vi "PicoScope2000GetTimebase2.vi"(4 "Number of Samples":u32, 6 "Memory Segment":u32, 7 "Acquisition Settings":T2 {"postTriggerSamples" format="%_6p"; "preTriggerSamples" format="%_6p"}, 10 "handle in":i16, 11 "error in (no error)":errorcluster) -> (2 "handle out":i16, 3 "error out":errorcluster, 5 "Properties Panel":T1 {"Max Total Capture Time Available (sec)" format="%.3p"; "Sample Frequency" format="%.3p"; "Sample Rate" format="%.3p"; "Max Samples Available" format="%.3p"; "Total Capture Time (sec)" format="%.3p"})   [LabVIEW 2009]
uses:
  ps2000.dll
  shared/Acquisition Settings.ctl
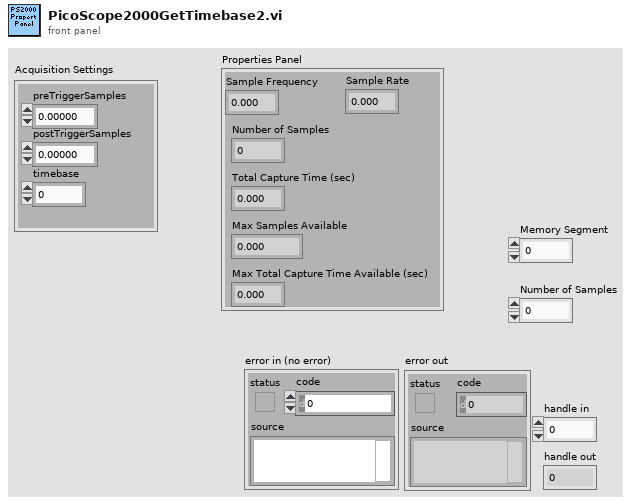
[diagram p1: front panel]
types:
  T1 = cluster{"Sample Frequency":sgl, "Sample Rate":sgl, "Max Samples Available":i32, "Number of Samples":u32, "Total Capture Time (sec) ":sgl, "Max Total Capture Time Available (sec)":sgl}
  T2 = typedef "Acquisition Settings.ctl" = cluster{"preTriggerSamples":u64, "postTriggerSamples":u64, "timebase":u32}
  T3 = cluster{sgl, sgl, "maxSamples":i32, "Number of Samples":u32, sgl, sgl}
  T4 = cluster{sgl, sgl, "max_sample":i32, "Number of Samples":u32, sgl, sgl}
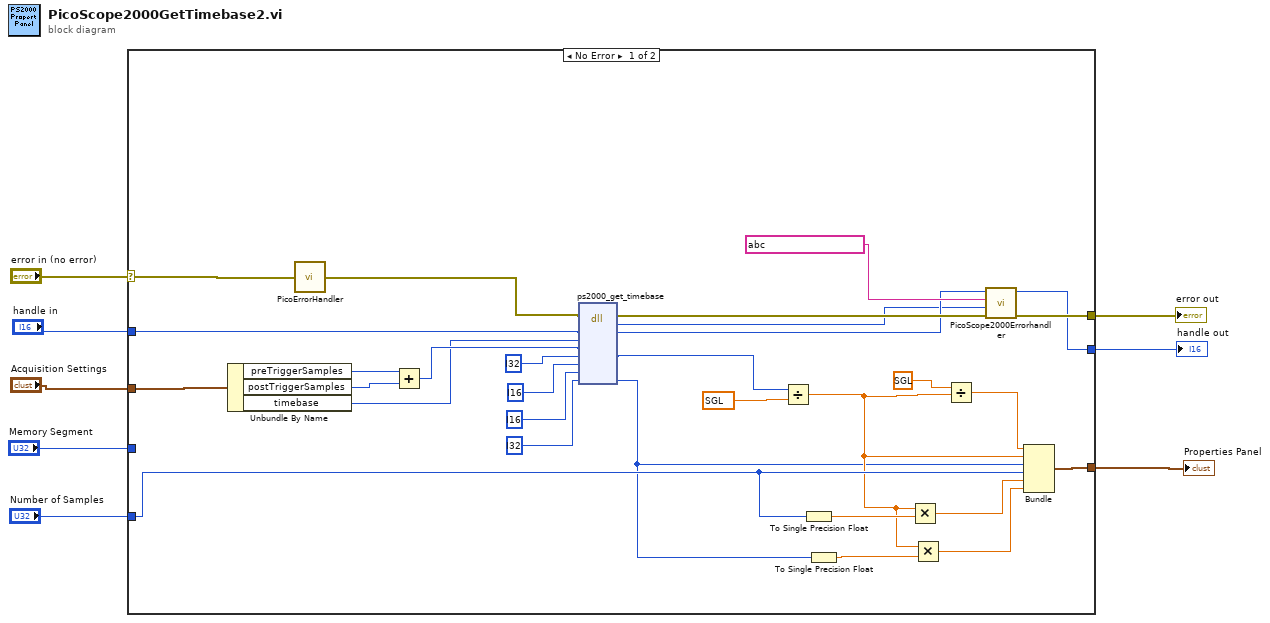
[diagram p0: block diagram]
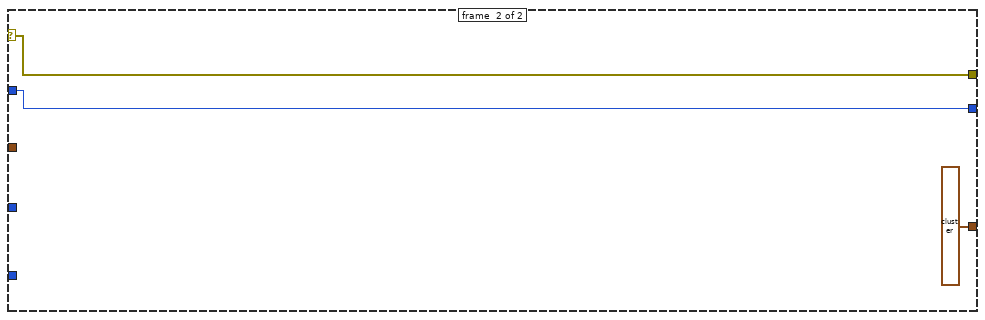
[diagram p2: hidden frame]
diagram:
  n1 = case shown="No Error" "error in (no error)" {
    selector: "error in (no error)" -> [w35 w41]
    tunnel: [w12 w41] -> w8
    tunnel: [w11 w40] -> w7
    tunnel: "Memory Segment" -> [_ _]
    tunnel: "Number of Samples" -> [w31 _]
    tunnel: "handle in" -> [w22 w40]
    tunnel: "Acquisition Settings" -> [w34 _]
    tunnel: [w28 T3 ?] -> w1
    frame #0 {
      n2 = Unbundle By Name(w34) -> ("preTriggerSamples"=w36:u64, "postTriggerSamples"=w37:u64, "timebase"=w20:u32)
      n3 = call "PicoErrorHandler.vi"("error in"=w35) -> ("error out"=w23:errorcluster)
      n4 = Add(x=w36, y=w37) -> (x+y=w21:u64)
      n5 = dll-call lib="PS2000.dll" fn="ps2000_get_timebase"(error in=w23, "handle"=w22, "timebase"=w20, "no_of_samples"=w21, "time_interval_ms"=i32 ?, "time_units"=i16 ?, "oversample"=i16 ?, "max_sample"=i32 ? ("maxSamples")) -> (error out=w13:errorcluster, "return type"=w9:i16, "handle"=w10:i16, "time_interval_ms"=w15:i32, "max_sample"=w24:i32)  [unwired: 6 in, 1 out]
      n6 = Divide(x=w15, y=sgl ?) -> (x/y=w27:sgl)
      n7 = To Single Precision Float(number=w31) -> (single precision float=w33:sgl)
      n8 = To Single Precision Float(number=w24) -> (single precision float=w30:sgl)
      n9 = Multiply(x=w27, y=w33) -> (x*y=w32:sgl)
      n10 = Multiply(x=w27, y=w30) -> (x*y=w29:sgl)
      n11 = Divide(x=sgl ?, y=w27) -> (x/y=w25:sgl)
      n12 = call "PicoScope2000Errorhandler.vi"("Handle in"=w10, "API function"=string ? ("source"), "Return"=w9, "error in (no error)"=w13) -> ("Handle out"=w11:i16, "error out"=w12:errorcluster)  [unwired: 5 in]
      n13 = Bundle(w25, w27, "max_sample"=w24, "Number of Samples"=w31, w32, w29) -> (w28:T4)  [unwired: 1 in]
    }
    frame #1 {
    }
  }
  "error out" <- w8
  "handle out" <- w7
  "Properties Panel" <- w1
